vi "Voorbeeld_Arrays.vi"() -> ()   [LabVIEW 2019]
panel:
  out "subarray":i32[](array[numeric])
  in  "index (row) 2":i32
  out "element":i32
  in  "disabled index (col)":i32
  in  "index (row)":i32
  out "size(s) 2":i32[](array[numeric])
  in  "Array 3":i32[][](array[numeric])=[[5, 2, 3], [1, 6, 4]]
  out "Array 2":bool[](array[boolean])
  in  "stop":bool
  out "size(s)":i32
  in  "Array":bool[](array[boolean])=[TRUE, TRUE, TRUE, FALSE, TRUE, FALSE, FALSE, FALSE, TRUE, TRUE]
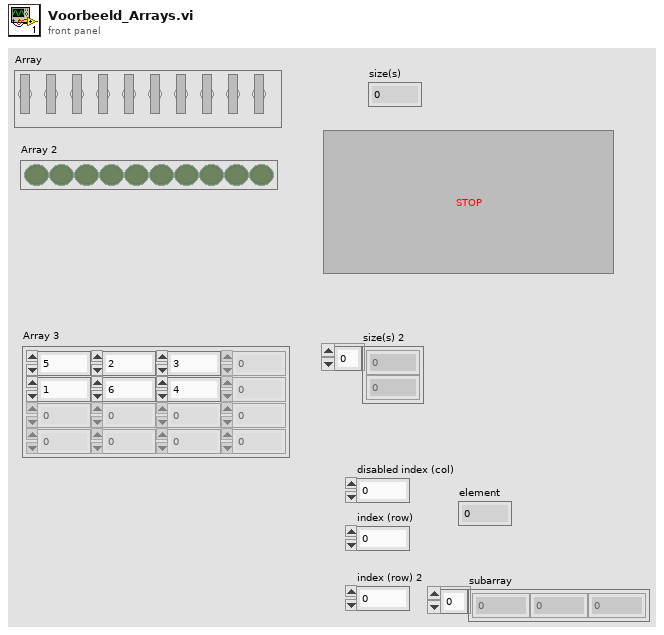
[diagram p1: front panel]
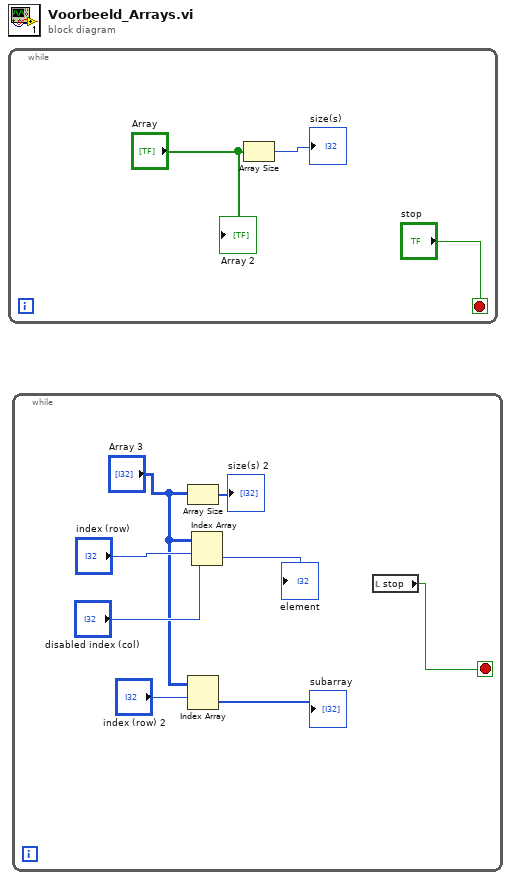
[diagram p0: block diagram]
diagram:
  n1 = while {
    stop <- "stop" stop-if-true
    n2 = Array Size(array="Array") -> (size(s)=→"size(s)":i32)
    "Array 2" <- "Array"
  }
  n3 = while {
    stop <- w11 stop-if-true
    n4 = Array Size(array="Array 3") -> (size(s)=→"size(s) 2":i32[])
    n5 = Index Array(array="Array 3", index (row)="index (row) 2") -> (element=→"subarray":i32[])  [unwired: 1 in]
    n6 = Index Array(array="Array 3", index (row)="index (row)", index (col)="disabled index (col)") -> (element=→"element":i32)
    n7 = local read "stop"() -> (w11:bool)
  }
